vi "CreateExerciseConfiguration.vi"(11 "Exericise Generation Array":bool[](array[boolean])) -> (3 "Exercise Configuration":T1)   [LabVIEW 2014]
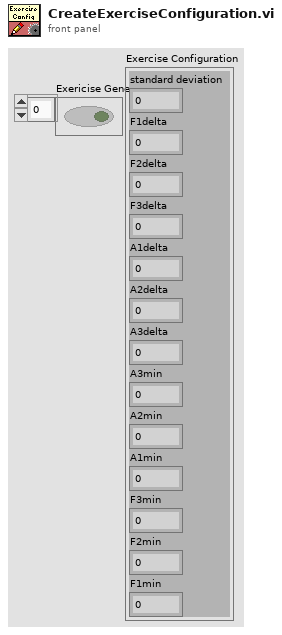
[diagram p1: front panel]
types:
  T1 = cluster{"standard deviation":dbl, "F1delta":dbl, "F2delta":dbl, "F3delta":dbl, "A1delta":dbl, "A2delta":dbl, "A3delta":dbl, "A3min":dbl, "A2min":dbl, "A1min":dbl, "F3min":dbl, "F2min":dbl, "F1min":dbl}
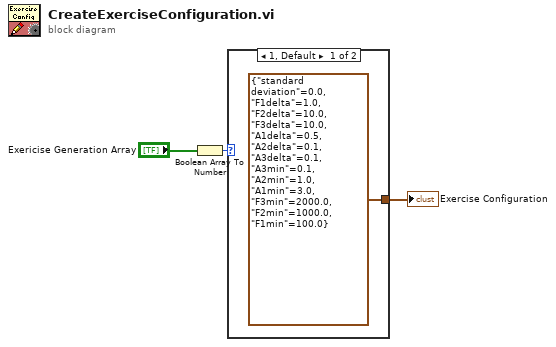
[diagram p0: block diagram]
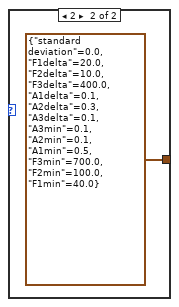
[diagram p2: hidden frame]
diagram:
  n1 = Boolean Array To Number(Boolean array="Exericise Generation Array") -> (number=w2:u32)
  n2 = case shown="1, Default" w2 {
    tunnel: [T1 {"standard deviation"=0.0, "F1delta"=1.0, "F2delta"=10.0, "F3delta"=10.0, "A1delta"=0.5, "A2delta"=0.1, "A3delta"=0.1, "A3min"=0.1, "A2min"=1.0, "A1min"=3.0, "F3min"=2000.0, "F2min"=1000.0, "F1min"=100.0} ("F & A") T1 {"standard deviation"=0.0, "F1delta"=20.0, "F2delta"=10.0, "F3delta"=400.0, "A1delta"=0.1, "A2delta"=0.3, "A3delta"=0.1, "A3min"=0.1, "A2min"=0.1, "A1min"=0.5, "F3min"=700.0, "F2min"=100.0, "F1min"=40.0} ("F & A")] -> w1
    frame 1, Default {
    }
    frame 2 {
    }
  }
  "Exercise Configuration" <- w1
